vi "Handle Depth Image.vi"(4 "queue in":refnum<queue>, 5 "Event Data":cluster{"sender":refnum<k24>, "e":refnum<k24>}, 6 "Control Ref":refnum<k24>, 7 "Event Common Data":T1) -> ()   [LabVIEW 2011]
uses:
  Microsoft.Kinect
  <vilib>/vision/Image Controls.llb/IMAQ Image.ctl
  Kinect/Kinect Global Status.vi
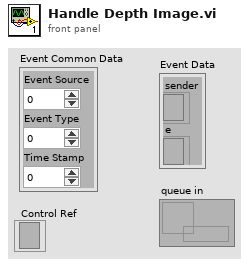
[diagram p1: front panel]
types:
  T1 = cluster{"Event Source":i32, "Event Type":u32, "Time Stamp":u32}
  T2 = typedef "Image Type" = u32
  T3 = typedef "IMAQ Image.ctl" = refnum<image>
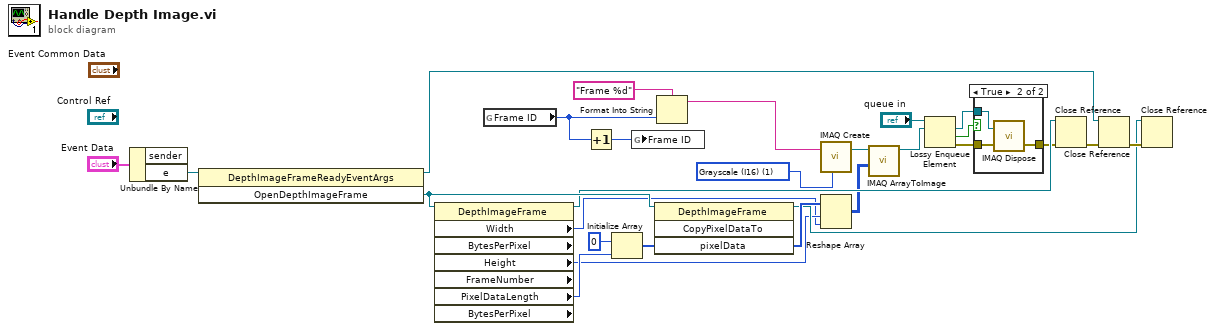
[diagram p0: block diagram]
diagram:
  w21 = T2 1 items=["Grayscale (U8)", "Grayscale (I16)", "Grayscale (SGL)", "Complex (CSG)", "RGB (U32)", "HSL (U32)", "RGB (U64)", "Grayscale (U16)"] ("Image Type")
  n1 = Unbundle By Name("Event Data") -> ("e"=w27:refnum<k24>)  [unwired: 1 out]
  n2 = invoke class="DepthImageFrameReadyEventArgs" method="OpenDepthImageFrame"(reference=w27) -> (reference out=w16:refnum<k24>, "OpenDepthImageFrame"=w26:refnum<k24>)  [unwired: 2 in, 1 out]
  n3 = property on="Property Node" class="DepthImageFrame" props=["Width", "BytesPerPixel", "Height", "FrameNumber", "PixelDataLength", "BytesPerPixel"](reference=w26) -> (reference out=w18:refnum<k24>, "Width"=w6:i32, "Height"=w7:i32, "PixelDataLength"=w19:i32)  [unwired: 1 in, 4 out]
  n4 = global read "Kinect Global Status.vi" "Frame ID"() -> (w2:i32)
  n5 = Increment(x=w2) -> (x+1=w1:i32)
  n6 = Initialize Array(i16 0 ("element"), w19) -> (w25:i16[])
  n7 = global write "Kinect Global Status.vi" "Frame ID"(w1) -> ()
  n8 = invoke class="DepthImageFrame" method="CopyPixelDataTo"(reference=w26, "pixelData"=w25) -> (reference out=w8:refnum<k24>, "pixelData"=w20:i16[])  [unwired: 2 in, 2 out]
  n9 = Format Into String(format string="Frame %d" ("Image Name"), w2) -> (resulting string=w3:string)  [unwired: 2 in, 1 out]
  n10 = call "IMAQ Create"("Image Name"=w3, "Image Type"=w21) -> ("New Image"=w22:T3)  [unwired: 3 in, 1 out]
  n11 = Reshape Array(w20, w7, w6) -> (w5:i16[][])
  n12 = call "IMAQ ArrayToImage"("Image Pixels (I16)"=w5, "Image"=w22) -> ("Image Out"=w14:T3)  [unwired: 8 in, 1 out]
  n13 = Lossy Enqueue Element(queue="queue in", element=w14) -> (overflow element=w10:T3, overflow?=w12:bool, error out=w11:errorcluster)  [unwired: 1 in, 1 out]
  n14 = case shown="True" w12 {
    tunnel: w11 -> [w28 w31]
    tunnel: [w28 w30] -> w15
    tunnel: w10 -> [_ w29]
    frame False {
    }
    frame True {
      n15 = call "IMAQ Dispose"("Image"=w29, "error in (no error)"=w31) -> ("error out"=w30:errorcluster)  [unwired: 4 in]
    }
  }
  n16 = Close Reference(reference=w18, error in (no error)=w15) -> (error out=w17:errorcluster)
  n17 = Close Reference(reference=w16, error in (no error)=w17) -> (error out=w9:errorcluster)
  n18 = Close Reference(reference=w8, error in (no error)=w9) -> ()  [unwired: 1 out]
